vi "TAT_Com_PLC.vi"() -> ()   [LabVIEW 2017]
uses:
  <vilib>/NI/Modbus Library/API/Wrapper/Create TCP Master.vi
  Global/Global 1.vi
  <vilib>/NI/Modbus Library/API/Master/Modbus Master.lvclass
  <vilib>/NI/Modbus Library/API/Wrapper/API Main.lvlib
panel:
  out "error out":errorcluster
  out "register values":u16[](array[numeric])
  out "Array":i32[](array[numeric])
  out "PLC STATUS":bool
  in  "error in":errorcluster
  in  "stop":bool
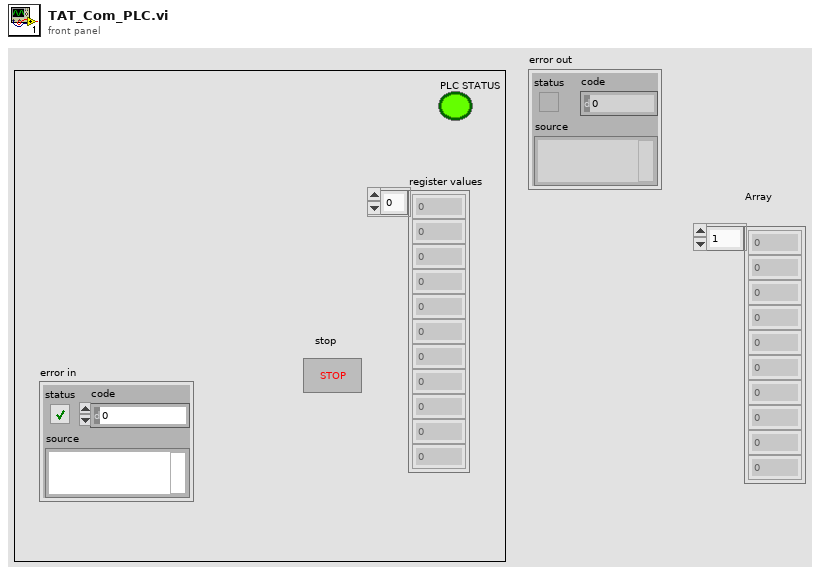
[diagram p1: front panel]
types:
  T1 = enum32{"invalid app kind", "Development System", "Run Time System", "Student Edition", "Embedded LabVIEW", "Evaluation", "Custom"}
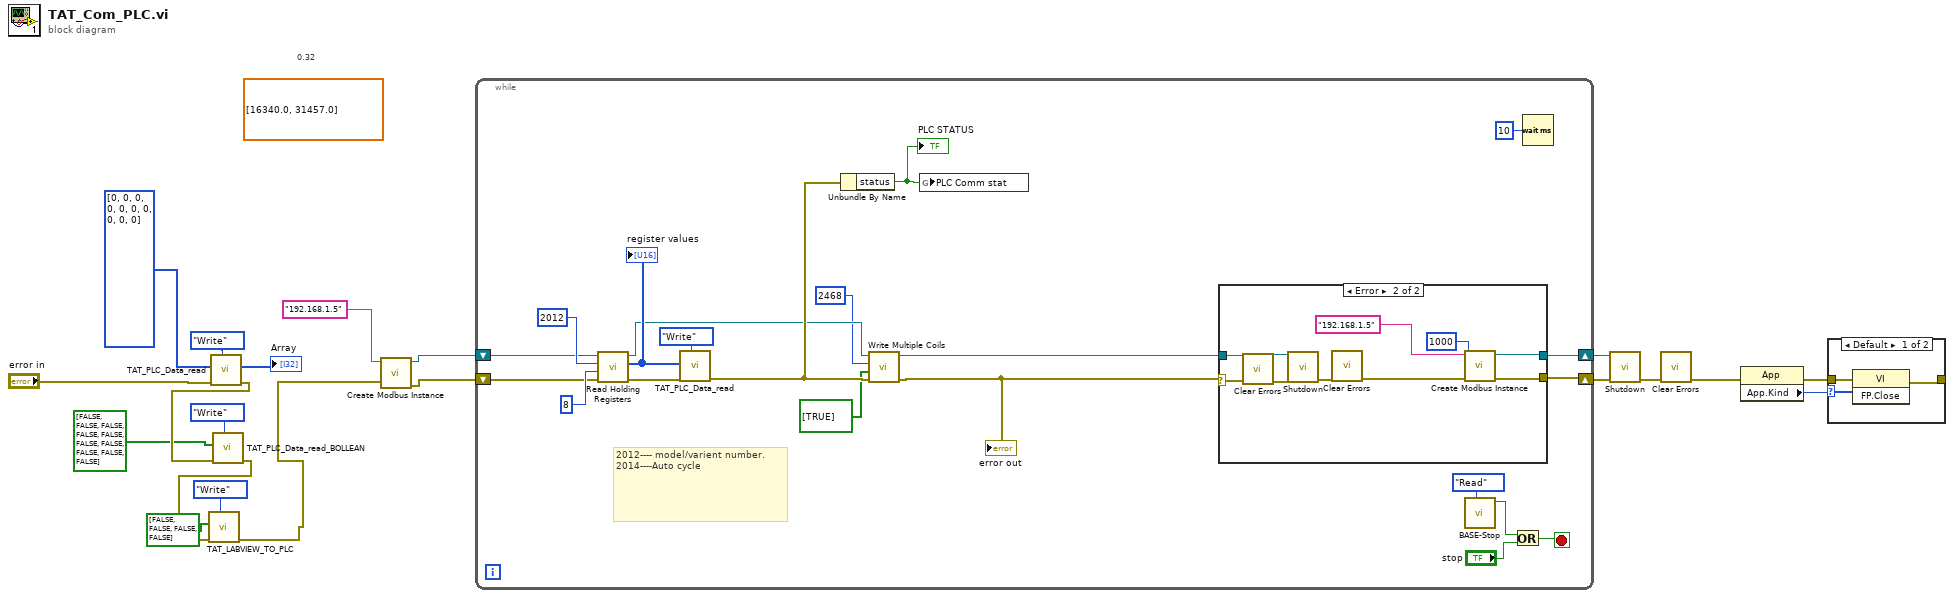
[diagram p0: block diagram]
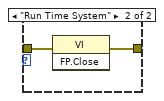
[diagram p3: hidden frame]
diagram:
  (unwired) dbl[] [16340.0, 31457.0] ("register values")
  # "0.32"
  n1 = call "TAT_PLC_Data_read.vi"("Enum"=enum16{"Read", "Write"}."Write", "error in (no error)"="error in", "Array"=i64[] [0, 0, 0, 0, 0, 0, 0, 0, 0, 0] ("Array 3")) -> ("error out"=w8:errorcluster, "Array 2"=→"Array":u16[])  [unwired: 7 in]
  n2 = call "TAT_PLC_Data_read_BOLLEAN.vi"("Enum"=enum16{"Read", "Write"}."Write", "error in (no error)"=w8, "Array"=bool[] [FALSE, FALSE, FALSE, FALSE, FALSE, FALSE, FALSE, FALSE, FALSE, FALSE]) -> ("error out"=w4:errorcluster)  [unwired: 7 in, 1 out]
  n3 = call "TAT_LABVIEW_TO_PLC.vi"("Enum"=enum16{"Read", "Write"}."Write", "error in (no error)"=w4, "Array"=bool[] [FALSE, FALSE, FALSE, FALSE]) -> ("error out"=w5:errorcluster)  [unwired: 7 in, 1 out]
  n4 = call-poly <vilib>:"Create Modbus Instance.vi"("error in"=w5, "address"="192.168.1.5") -> ("error out"=w15:errorcluster, "TCP master instance"=w14:refnum<class "Modbus Master.lvclass">)  [unwired: 8 in]
  n5 = while {
    shift-right: [w39] -> w19
    shift-left: w14 -> [w34]
    shift-right: [w38] -> w18
    shift-left: w15 -> [w35]
    stop <- w40 stop-if-true
    # "2012---- model/varient number.\n2014----Auto cycle"
    n6 = call-dynamic "Read Holding Registers.vi"("error in"=w35, "number of inputs"=u16 8 ("number of register"), "starting address"=u16 2012, "Modbus master in"=w34) -> ("error out"=w30:errorcluster, "register values"=w32:u16[], "Modbus master out"=w24:refnum<class "Modbus Master.lvclass">)  [unwired: 5 in]
    "register values" <- w32
    n7 = call "TAT_PLC_Data_read.vi"("Enum"=enum16{"Read", "Write"}."Write", "error in (no error)"=w30, "Array"=w32) -> ("error out"=w26:errorcluster)  [unwired: 7 in, 1 out]
    n8 = Unbundle By Name(w26) -> ("status"=w27:bool)
    "PLC STATUS" <- w27
    n9 = call-dynamic "Write Multiple Coils.vi"("error in"=w26, "coils to write"=bool[] [TRUE], "starting address"=u16 2468, "Modbus master in"=w24) -> ("error out"=w25:errorcluster, "Modbus master out"=w23:refnum<class "Modbus Master.lvclass">)  [unwired: 6 in]
    "error out" <- w25
    n10 = global write "Global 1.vi" "PLC Comm stat"(w27) -> ()
    n11 = case shown="Error" w25 {
      selector: w25 -> [w42 w52]
      tunnel: w23 -> [w43 w50]
      tunnel: [w43 w46] -> w39
      tunnel: [w42 w45] -> w38
      frame No Error {
      }
      frame Error {
        n12 = call <vilib>:"Clear Errors.vi"("error in (no error)"=w52) -> ("error out"=w51:errorcluster)  [unwired: 5 in, 1 out]
        n13 = call-dynamic "Shutdown.vi"("error in"=w51, "Modbus master in"=w50) -> ("error out"=w49:errorcluster)  [unwired: 9 in]
        n14 = call <vilib>:"Clear Errors.vi"("error in (no error)"=w49) -> ("error out"=w47:errorcluster)  [unwired: 5 in, 1 out]
        n15 = call-poly <vilib>:"Create Modbus Instance.vi"("error in"=w47, "connect timeout ms"=1000, "address"="192.168.1.5") -> ("error out"=w45:errorcluster, "TCP master instance"=w46:refnum<class "Modbus Master.lvclass">)  [unwired: 7 in]
      }
    }
    n16 = call "BASE-Stop.vi"("Enum"=enum16{"Read", "Write"}."Read") -> ("Stop"=w28:bool)  [unwired: 10 in]
    n17 = Or(x=w28, y="stop") -> (x .or. y?=w40:bool)
    n18 = Wait (ms)(milliseconds to wait=u32 10) -> ()  [unwired: 1 out]
  }
  n19 = call-dynamic "Shutdown.vi"("error in"=w18, "Modbus master in"=w19) -> ("error out"=w2:errorcluster)  [unwired: 9 in]
  n20 = call <vilib>:"Clear Errors.vi"("error in (no error)"=w2) -> ("error out"=w1:errorcluster)  [unwired: 5 in, 1 out]
  n21 = property class="App"(error in=w1) -> (error out=w16:errorcluster, "App.Kind"=w17:T1)  [unwired: 1 in, 1 out]
  n22 = case shown="Default" w17 {
    tunnel: w16 -> [w54 w56]
    tunnel: [w53 w55] -> _
    frame Default {
      n23 = invoke class="VI" method="FP.Close"(error in=w54) -> (error out=w53:errorcluster)  [unwired: 2 in, 2 out]
    }
    frame "Run Time System" {
      n24 = invoke class="VI" method="FP.Close"(error in=w56) -> (error out=w55:errorcluster)  [unwired: 2 in, 2 out]
    }
  }
